vi "String to DAQmx PhysCh.vi"(1 "Channel String":string, 2 "Resource Name":string) -> (0 "DAQmx Physical Channels":string)   [LabVIEW 2020, in "BNT_ULx.lvlib" / "BNT_ULx-MCSV.lvclass"]
doc: "Create DAQmx Physical Channel string from ini-file item."
uses:
  BNT_ULx-MCSV.lvclass
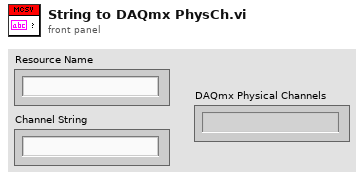
[diagram p1: front panel]
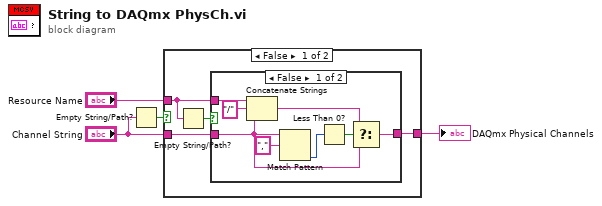
[diagram p0: block diagram]
diagram:
  n1 = Empty String/Path?(string/path="Channel String") -> (empty?=w2:bool)
  n2 = case shown="False" w2 {
    tunnel: "Channel String" -> [w8 _]
    tunnel: [w6 _] -> w4
    tunnel: "Resource Name" -> [w5 _]
    frame False {
      n3 = Empty String/Path?(string/path=w5) -> (empty?=w7:bool)
      n4 = case shown="False" w7 {
        tunnel: w5 -> [w12 _]
        tunnel: w8 -> [w11 w17]
        tunnel: [w9 w17] -> w6
        frame False {
          n5 = Concatenate Strings(w12, "/" ("string"), w11) -> (w13:string)
          n6 = Match Pattern(string=w11, regular expression=",") -> (offset past match=w15:i32)  [unwired: 1 in, 3 out]
          n7 = Less Than 0?(x=w15) -> (x < 0?=w16:bool)
          n8 = Select(t=w13, s=w16, f=w11) -> (s? t:f=w9:string)
        }
        frame True {
        }
      }
    }
    frame True {
    }
  }
  "DAQmx Physical Channels" <- w4
